vi "Quinn's second method interpolation.vi"(8 "FFT Imm":dbl[](array[numeric]), 11 "FFT real":dbl[](array[numeric])) -> (2 "Index Bin":dbl)   [LabVIEW 2014]
panel:
  out "max index(es)":i32
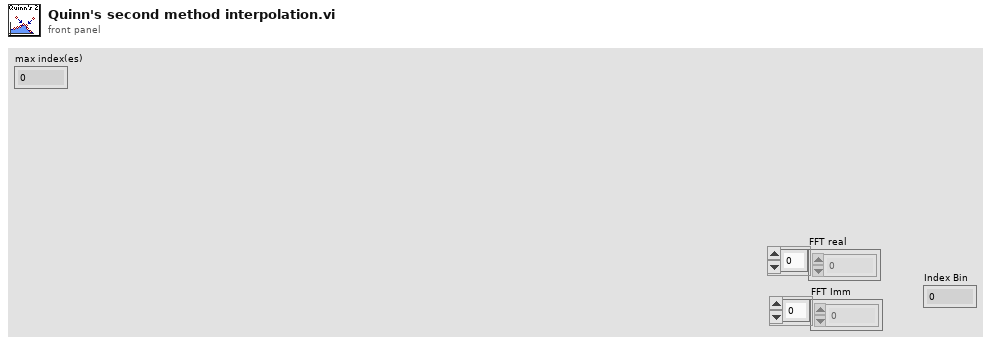
[diagram p1: front panel]
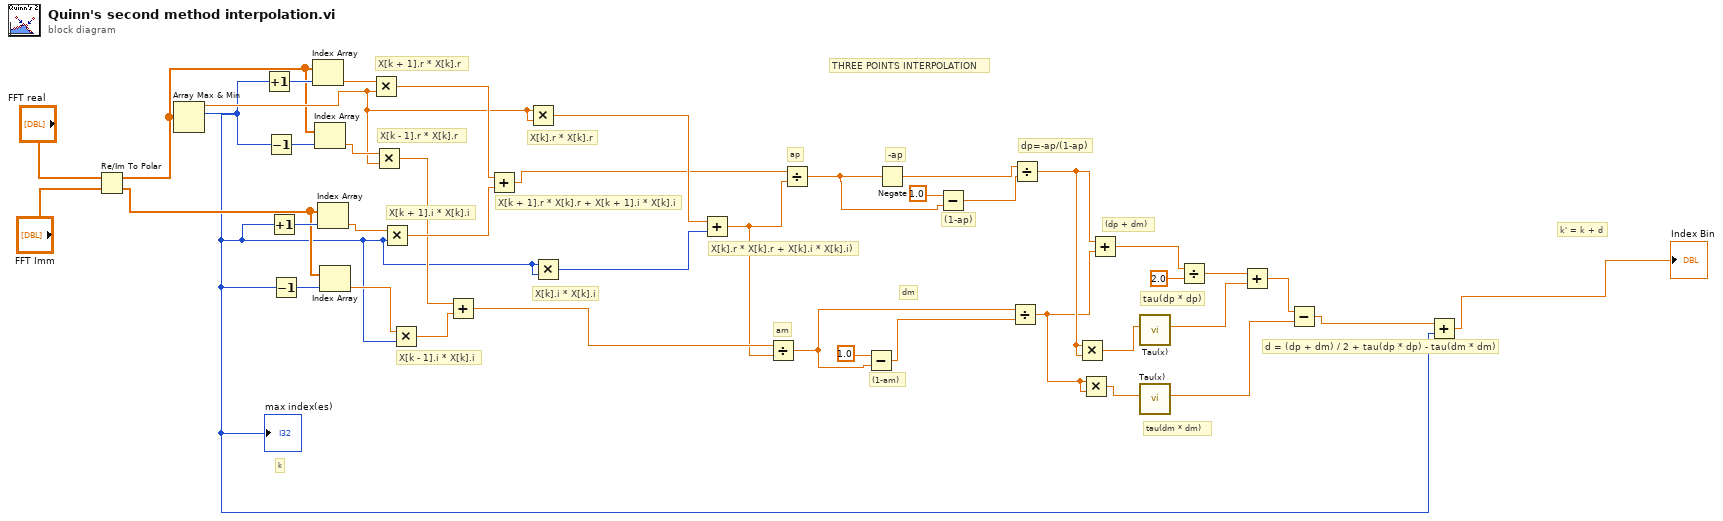
[diagram p0: block diagram]
diagram:
  # "THREE POINTS INTERPOLATION"
  # "k' = k + d"
  # "d = (dp + dm) / 2 + tau(dp * dp) - tau(dm * dm)"
  # "tau(dm * dm)"
  # "tau(dp * dp)"
  # "(dp + dm)"
  # "k"
  # "dm"
  # "(1-am)"
  # "am"
  # "X[k - 1].r * X[k].r"
  # "X[k - 1].i * X[k].i"
  # "dp=-ap/(1-ap)"
  # "(1-ap)"
  # "-ap"
  # "ap"
  # "X[k].r * X[k].r + X[k].i * X[k].i)"
  # "X[k + 1].r * X[k].r + X[k + 1].i * X[k].i"
  # "X[k].r * X[k].r"
  # "X[k].i * X[k].i"
  # "X[k + 1].i * X[k].i"
  # "X[k + 1].r * X[k].r"
  n1 = Re/Im To Polar(2:"FFT Imm", 3:"FFT real") -> (0:w16:dbl[], 1:w17:dbl[])
  n2 = Array Max & Min(array=w17) -> (max value=w25:dbl, max index (indices)=w2:i32)  [unwired: 2 out]
  "max index(es)" <- w2
  n3 = Increment(x=w2) -> (x+1=w42:i32)
  n4 = Decrement(x=w2) -> (x-1=w41:i32)
  n5 = Increment(x=w2) -> (x+1=w39:i32)
  n6 = Decrement(x=w2) -> (x-1=w40:i32)
  n7 = Index Array(array=w17, index=w42) -> (element=w38:dbl)
  n8 = Index Array(array=w17, index=w41) -> (element=w26:dbl)
  n9 = Index Array(array=w16, index=w39) -> (element=w37:dbl)
  n10 = Index Array(array=w16, index=w40) -> (element=w27:dbl)
  n11 = Multiply(x=w38, y=w25) -> (x*y=w36:dbl)
  n12 = Multiply(x=w26, y=w25) -> (x*y=w23:dbl)
  n13 = Multiply(x=w37, y=w2) -> (x*y=w35:dbl)
  n14 = Multiply(x=w27, y=w2) -> (x*y=w24:dbl)
  n15 = Add(x=w23, y=w24) -> (x+y=w22:dbl)
  n16 = Add(x=w36, y=w35) -> (x+y=w32:dbl)
  n17 = Multiply(x=w25, y=w25) -> (x*y=w33:dbl)
  n18 = Multiply(x=w2, y=w2) -> (x*y=w34:i32)
  n19 = Add(x=w33, y=w34) -> (x+y=w21:dbl)
  n20 = Divide(x=w22, y=w21) -> (x/y=w19:dbl)
  n21 = Divide(x=w32, y=w21) -> (x/y=w30:dbl)
  n22 = Subtract(x=1.0, y=w19) -> (x-y=w18:dbl)
  n23 = Negate(x=w30) -> (-x=w29:dbl)
  n24 = Subtract(x=1.0, y=w30) -> (x-y=w28:dbl)
  n25 = Divide(x=w19, y=w18) -> (x/y=w5:dbl)
  n26 = Divide(x=w29, y=w28) -> (x/y=w8:dbl)
  n27 = Multiply(x=w8, y=w8) -> (x*y=w9:dbl)
  n28 = Multiply(x=w5, y=w5) -> (x*y=w6:dbl)
  n29 = Add(x=w8, y=w5) -> (x+y=w13:dbl)
  n30 = call "Tau(x).vi"("X"=w9) -> ("Tau"=w10:dbl)  [unwired: 10 in]
  n31 = call "Tau(x).vi"("X"=w6) -> ("Tau"=w4:dbl)  [unwired: 10 in]
  n32 = Divide(x=w13, y=2.0) -> (x/y=w11:dbl)
  n33 = Add(x=w11, y=w10) -> (x+y=w7:dbl)
  n34 = Subtract(x=w7, y=w4) -> (x-y=w3:dbl)
  n35 = Add(x=w3, y=w2) -> (x+y=→"Index Bin":dbl)
